vi "Image Get.vi"(8 "error in":errorcluster, 11 "Image Path":path=path "F:/designer/LabView/pictures/cells/IMG00028.JPG") -> (0 "error out":errorcluster, 1 "Image Resolution":sgl[][](array[numeric]), 2 "cell para":sgl[][](array[numeric]), 3 "Image Out":T1, 5 "Number of Matches":sgl)   [LabVIEW 2016]
uses:
  <vilib>/vision/Image Controls.llb/IMAQ Image.ctl
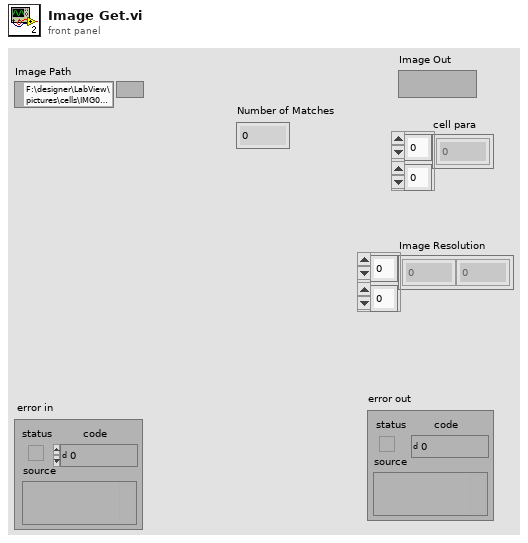
[diagram p1: front panel]
types:
  T1 = typedef "IMAQ Image.ctl" = refnum<image>
  T2 = cluster{"Position":cluster{"x":sgl, "y":sgl}, "Angle":sgl, "Scale":sgl, "Score":sgl, "Bounding Box":cluster{"x":sgl, "y":sgl}[]}[]
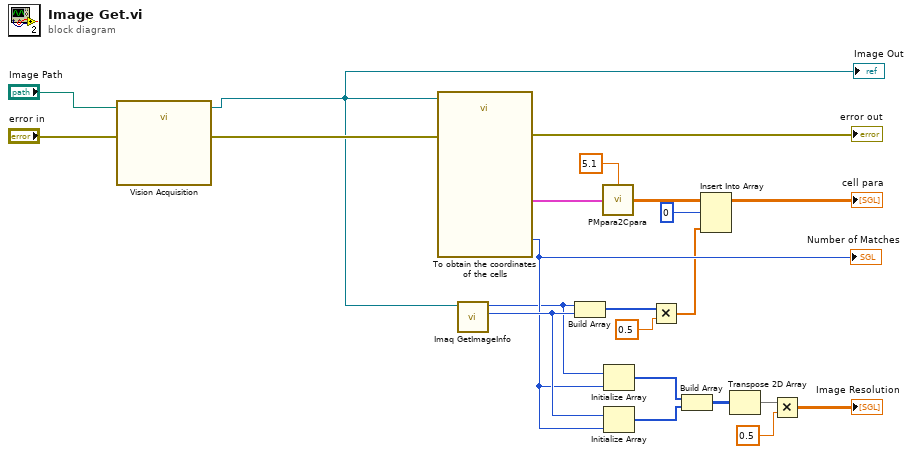
[diagram p0: block diagram]
diagram:
  n1 = call "Vision Acquisition"("Image Path"="Image Path", "error in"="error in") -> ("Image Out"=w1:T1, "error out"=w2:errorcluster)  [unwired: 24 in]
  "Image Out" <- w1
  n2 = call "To obtain the coordinates of the cells"("Image In"=w1, "error in"=w2) -> ("Matches (Pattern Matching)"=w6:T2, "Number of Matches (Pattern Matching)"=w15:i32, "error out"=→"error out":errorcluster)  [unwired: 21 in, 2 out]
  "Number of Matches" <- w15
  n3 = call "Imaq GetImageInfo"("Image"=w1) -> ("Y Resolution"=w16:i32, "X Resolution"=w14:i32)  [unwired: 3 in, 6 out]
  n4 = Build Array(w14, w16) -> (w11:i32[])
  n5 = call "PMpara2Cpara.vi"("PM para"=w6, "Resolution multiple"=5.1) -> ("cell para"=w9:sgl[][])
  n6 = Initialize Array(w14, w15) -> (w17:i32[])
  n7 = Initialize Array(w16, w15) -> (w18:i32[])
  n8 = Multiply(x=w11, y=0.5) -> (x*y=w13:dbl[])
  n9 = Build Array(w17, w18) -> (w19:i32[][])
  n10 = Insert Into Array(array=w9, index (row)=0 ("索引 (行)"), new element=w13) -> (→"cell para":sgl[][])  [unwired: 1 in]
  n11 = Transpose 2D Array(2D array=w19) -> (transposed array=w21:i32[][])
  n12 = Multiply(x=w21, y=0.5) -> (x*y=→"Image Resolution":dbl[][])
